vi "Read.vi"(8 "error in (no error)":errorcluster, 11 "Sparkfun Atomic IMU in":refnum<class "Sparkfun Atomic IMU.lvclass">) -> (0 "error out":errorcluster, 1 "Gyros Data":T1, 2 "Accelerometer Data":T2, 3 "Sparkfun Atomic IMU out":refnum<class "Sparkfun Atomic IMU.lvclass">)   [LabVIEW 2019, in "Sparkfun Atomic IMU.lvclass"]
doc: "Reads accelerometer data, gyros data from sensor."
uses:
  Sparkfun Atomic IMU.lvclass
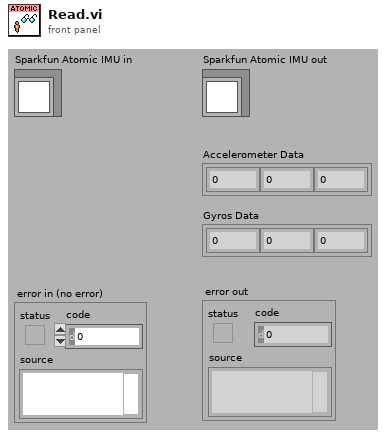
[diagram p1: front panel]
types:
  T1 = cluster{"Pitch (deg/s)":dbl, "Roll (deg/s)":dbl, "Yaw (deg/s)":dbl}
  T2 = cluster{"Accel_X (g)":dbl, "Accel_Y (g)":dbl, "Accel_Z (g)":dbl}
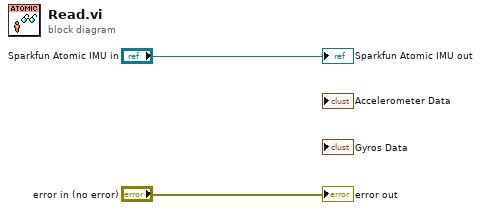
[diagram p0: block diagram]
diagram:
  "Sparkfun Atomic IMU out" <- "Sparkfun Atomic IMU in"
  "error out" <- "error in (no error)"
